vi "Get Value list.vi"(8 "error in (no error)":errorcluster, 10 "Indice de fila":i32, 11 "Nestle Actor in":refnum<class "Nestle Actor.lvclass">) -> (0 "error out":errorcluster, 3 "Nestle Actor out":refnum<class "Nestle Actor.lvclass">)   [LabVIEW 2020, in "Nestle Actor.lvlib" / "Nestle Actor.lvclass"]
uses:
  Nestle Actor.lvclass
  C:/Program Files (x86)/National Instruments/LabVIEW 2020/vi.lib/ActorFramework/Actor/Actor.lvclass
  <vilib>/ActorFramework/Actor/Actor.lvclass/Actor.ctl
  Nestle Actor.lvclass/Nestle Actor.ctl
  UI Actor Messages/Update Values Msg/Update Values Msg.lvclass/Update Values Msg.ctl
  <vilib>/ActorFramework/Message Enqueuer/Message Enqueuer.lvclass/Message Enqueuer.ctl
  <vilib>/ActorFramework/Message Enqueuer/Enqueue.vi
  UI Actor Messages/Update Values Msg/Update Values Msg.lvclass
  C:/Program Files (x86)/National Instruments/LabVIEW 2020/vi.lib/ActorFramework/Message/Message.lvclass
  <vilib>/ActorFramework/Message Priority Queue/Priority Enqueue.vi
  <vilib>/ActorFramework/Actor/Actor.lvclass
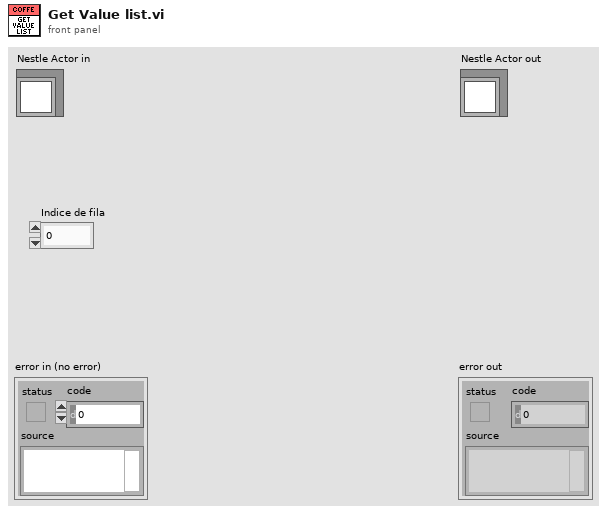
[diagram p1: front panel]
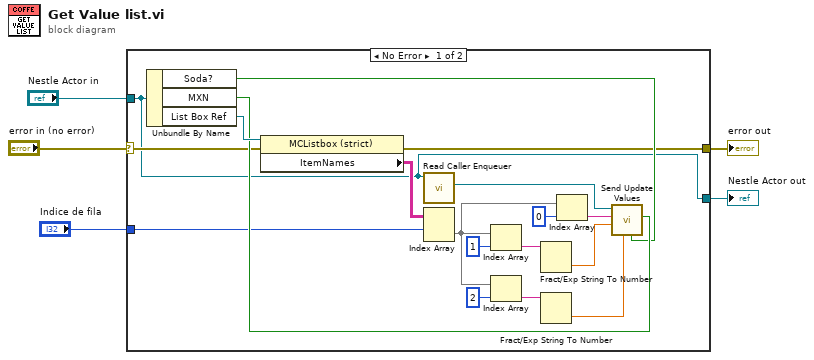
[diagram p0: block diagram]
diagram:
  n1 = case shown="No Error" "error in (no error)" {
    selector: "error in (no error)" -> [w9 w25]
    tunnel: [w8 w25] -> w4
    tunnel: [w6 w24] -> w2
    tunnel: "Nestle Actor in" -> [w6 w24]
    tunnel: "Indice de fila" -> [w7 _]
    frame No Error {
      n2 = Unbundle By Name(w6) -> ("Soda?"=w10:bool, "MXN"=w11:bool, "List Box Ref"=w23:refnum<vi>)
      n3 = property class="MCListbox (strict)"(reference=w23, error in=w9) -> (error out=w8:errorcluster, "ItemNames"=w22:string[][])  [unwired: 1 out]
      n4 = call <vilib>:"Read Caller Enqueuer.vi"("Actor"=w6) -> ("Caller Enqueuer"=w17:refnum<class "Message Enqueuer.lvclass">)  [unwired: 10 in]
      n5 = Index Array(array=w22, index (row)=w7) -> (element=w18:string[])  [unwired: 1 in]
      n6 = Index Array(array=w18, index=1 ("index (row)")) -> (element=w13:string)
      n7 = Index Array(array=w18, index=2 ("index (row)")) -> (element=w15:string)
      n8 = Fract/Exp String To Number(string=w13) -> (number=w12:dbl)  [unwired: 3 in, 1 out]
      n9 = Fract/Exp String To Number(string=w15) -> (number=w14:dbl)  [unwired: 3 in, 1 out]
      n10 = Index Array(array=w18, index=0 ("index (row)")) -> (element=w16:string)
      n11 = call "Send Update Values.vi"("MXN?"=w11, "Soda?"=w10, "Inventario"=w14, "Costo"=w12, "Producto"=w16, "Message Enqueuer"=w17) -> ()  [unwired: 4 in, 2 out]
    }
    frame Error {
    }
  }
  "error out" <- w4
  "Nestle Actor out" <- w2
